vi "Endpoint.vi"(7 "endpointOp":T3, 8 "element in":T4, 10 "parms in":T1={"subchannel"=0, "size (0)"=0, "abort (F)"=FALSE, "timeout"=-1, "ack id (0)"=0, "last elt? (F)"=FALSE, "valid? (T)"=FALSE, "GUID"=""}, 11 "channel in":T5) -> (0 "element out":T4, 2 "parms out":T2)   [LabVIEW 2019, in "MessengerM.lvlib"]
doc: "Reads a message from a MsgPipe Channel (blocks if empty, but not beyond the specified timeout)."
uses:
  <resource>/Channels/MessengerM/MessengerM.lvlib
  <resource>/Channels/MessengerM/ChannelOp.ctl
  <resource>/ChannelSupport/_ChannelSupport/_ChannelSupport.lvlib
  <resource>/Channels/MessengerM/EndpointOp.ctl
  <resource>/Channels/MessengerM/))Channel.ctl
  <resource>/Channels/MessengerM/Element.ctl
  <resource>/Channels/MessengerM/ParmsOut.ctl
  <resource>/Channels/MessengerM/ParmsIn.ctl
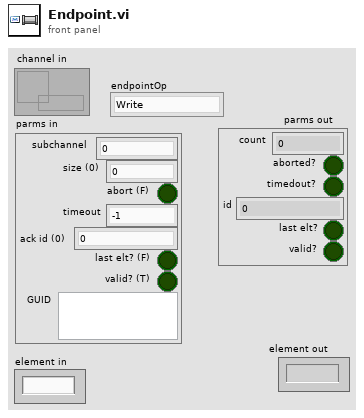
[diagram p1: front panel]
types:
  T1 = typedef "MessengerM.lvlib/ParmsIn.ctl" = cluster{"subchannel":i32, "size (0)":i32, "abort (F)":bool, "timeout":i32, "ack id (0)":u32, "last elt? (F)":bool, "valid? (T)":bool, "GUID":string}
  T2 = typedef "MessengerM.lvlib/ParmsOut.ctl" = cluster{"count":i32, "aborted?":bool, "timedout?":bool, "id":u32, "last elt?":bool, "valid?":bool}
  T3 = typedef "MessengerM.lvlib/EndpointOp.ctl" = enum16{"Write", "WriteAck", "WriteSync", "Read", "ReadAck"}
  T4 = typedef "MessengerM.lvlib/Element.ctl" = string
  T5 = typedef "MessengerM.lvlib/))Channel.ctl" = refnum<queue>
  T6 = typedef "MessengerM.lvlib/ChannelOp.ctl" = enum16{"init", "write", "read", "wreplace", "rreplace", "wrtAck", "rdAck", "rdAck2", "packet", "probe"}
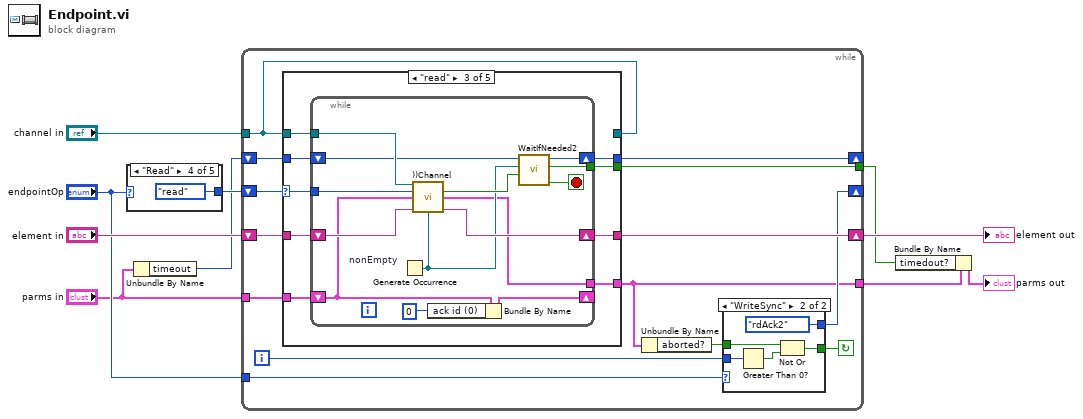
[diagram p0: block diagram]
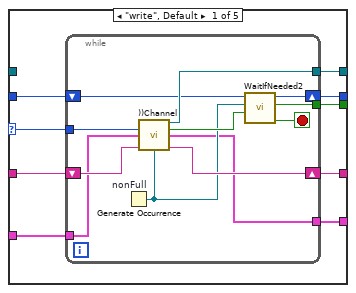
[diagram p2: hidden frame]
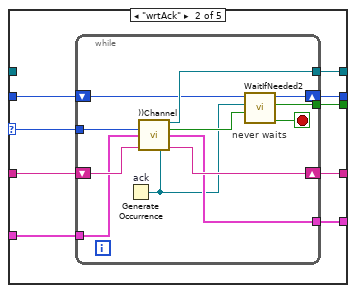
[diagram p3: hidden frame]
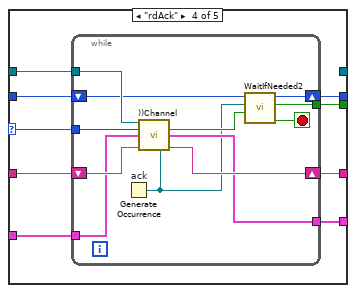
[diagram p4: hidden frame]
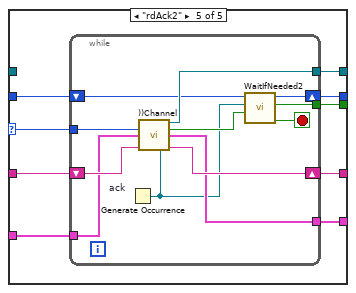
[diagram p5: hidden frame]
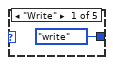
[diagram p7: hidden frame]
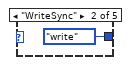
[diagram p8: hidden frame]
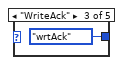
[diagram p9: hidden frame]
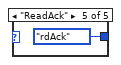
[diagram p10: hidden frame]
diagram:
  n1 = case shown="\"Read\"" "endpointOp" {
    tunnel: [ChannelOp."write" ("channelOp") ChannelOp."write" ("channelOp") ChannelOp."wrtAck" ("channelOp") ChannelOp."read" ("channelOp") ChannelOp."rdAck" ("channelOp")] -> w8
    frame "Write" {
    }
    frame "WriteSync" {
    }
    frame "WriteAck" {
    }
    frame "Read" {
    }
    frame "ReadAck" {
    }
  }
  n2 = Unbundle By Name("parms in") -> ("timeout"=w4:i32)
  n3 = while {
    tunnel: [w28] -> w1
    tunnel: "endpointOp" -> [w21]
    shift-right: [w23] -> _
    shift-left: w8 -> [w25]
    tunnel: "channel in" -> [w20]
    shift-right: [w29] -> w6
    shift-left: "element in" -> [w27]
    tunnel: "parms in" -> [w19]
    shift-right: [w18] -> _
    shift-left: w4 -> [w26]
    tunnel: [w17] -> w3
    i -> [w22]
    stop <- w24 continue-if-true
    n4 = case shown="\"read\"" w25 {
      selector: w25 -> [w34 w55 w76 w99 w120]
      tunnel: [w38 w59 w80 w103 w124] -> w29
      tunnel: [w37 w58 w79 w102 w123] -> w28
      tunnel: w27 -> [w36 w57 w78 w101 w122]
      tunnel: w26 -> [w35 w56 w77 w100 w121]
      tunnel: [w33 w54 _ _ w119] -> w20
      tunnel: w20 -> [_ _ w75 w98 _]
      tunnel: w19 -> [w30 w51 w72 w95 w118]
      tunnel: [w32 w53 w74 w97 w117] -> w18
      tunnel: [w31 w52 w73 w96 w116] -> w17
      frame "write", Default {
        n5 = while {
          tunnel: w34 -> [w49]
          tunnel: [w46] -> w37
          tunnel: [w47] -> w33
          shift-right: [w50] -> w38
          shift-left: w36 -> [w48]
          shift-right: [w41] -> w32
          shift-left: w35 -> [w44]
          tunnel: [w40] -> w31
          tunnel: w30 -> [w39]
          stop <- w45 stop-if-true
          n6 = Generate Occurrence "nonFull"() -> (w42:refnum<k4>)
          n7 = call <resource>:"))Channel.vi"("channelOp"=w49, "parms in"=w39, "element in"=w48, "nonfull/empty"=w42) -> ("channel out"=w47:T5, "wait"=w43:bool, "parms out"=w40:T2, "element out"=w50:T4)  [unwired: 6 in, 2 out]
          n8 = call <resource>:"WaitIfNeeded2.vi"("wait"=w43, "occ"=w42, "_timeout (ms) in"=w44) -> ("stop loop"=w45:bool, "timed out"=w46:bool, "_timeout (ms) out"=w41:i32)  [unwired: 6 in]
        }
      }
      frame "wrtAck" {
        n9 = while {
          tunnel: w55 -> [w70]
          tunnel: [w67] -> w58
          tunnel: [w68] -> w54
          shift-right: [w71] -> w59
          shift-left: w57 -> [w69]
          shift-right: [w63] -> w53
          shift-left: w56 -> [w65]
          tunnel: [w62] -> w52
          tunnel: w51 -> [w61]
          stop <- w66 stop-if-true
          # "never waits"
          n10 = Generate Occurrence "ack"() -> (w60:refnum<k4>)
          n11 = call <resource>:"))Channel.vi"("channelOp"=w70, "parms in"=w61, "element in"=w69, "ackOcc"=w60) -> ("channel out"=w68:T5, "wait"=w64:bool, "parms out"=w62:T2, "element out"=w71:T4)  [unwired: 6 in, 2 out]
          n12 = call <resource>:"WaitIfNeeded2.vi"("wait"=w64, "occ"=w60, "_timeout (ms) in"=w65) -> ("stop loop"=w66:bool, "timed out"=w67:bool, "_timeout (ms) out"=w63:i32)  [unwired: 6 in]
        }
      }
      frame "read" {
        n13 = while {
          tunnel: w76 -> [w93]
          tunnel: [w90] -> w79
          tunnel: w75 -> [w91]
          shift-right: [w94] -> w80
          shift-left: w78 -> [w92]
          shift-right: [w85] -> w74
          shift-left: w77 -> [w88]
          tunnel: [w84] -> w73
          shift-right: [w82] -> _
          shift-left: w72 -> [w83]
          stop <- w89 stop-if-true
          n14 = Generate Occurrence "nonEmpty"() -> (w86:refnum<k4>)
          n15 = call <resource>:"))Channel.vi"("channel in"=w91, "channelOp"=w93, "parms in"=w83, "element in"=w92, "nonfull/empty"=w86) -> ("wait"=w87:bool, "parms out"=w84:T2, "element out"=w94:T4)  [unwired: 5 in, 3 out]
          n16 = Bundle By Name(cluster=w83, "ack id (0)"=u32 0) -> (w82:T1)
          n17 = call <resource>:"WaitIfNeeded2.vi"("wait"=w87, "occ"=w86, "_timeout (ms) in"=w88) -> ("stop loop"=w89:bool, "timed out"=w90:bool, "_timeout (ms) out"=w85:i32)  [unwired: 6 in]
        }
      }
      frame "rdAck" {
        n18 = while {
          tunnel: w99 -> [w114]
          tunnel: [w111] -> w102
          tunnel: w98 -> [w112]
          shift-right: [w115] -> w103
          shift-left: w101 -> [w113]
          shift-right: [w107] -> w97
          shift-left: w100 -> [w109]
          tunnel: [w106] -> w96
          tunnel: w95 -> [w105]
          stop <- w110 stop-if-true
          n19 = Generate Occurrence "ack"() -> (w104:refnum<k4>)
          n20 = call <resource>:"))Channel.vi"("channel in"=w112, "channelOp"=w114, "parms in"=w105, "element in"=w113, "ackOcc"=w104) -> ("wait"=w108:bool, "parms out"=w106:T2, "element out"=w115:T4)  [unwired: 5 in, 3 out]
          n21 = call <resource>:"WaitIfNeeded2.vi"("wait"=w108, "occ"=w104, "_timeout (ms) in"=w109) -> ("stop loop"=w110:bool, "timed out"=w111:bool, "_timeout (ms) out"=w107:i32)  [unwired: 6 in]
        }
      }
      frame "rdAck2" {
        n22 = while {
          tunnel: w120 -> [w135]
          tunnel: [w132] -> w123
          tunnel: [w133] -> w119
          shift-right: [w136] -> w124
          shift-left: w122 -> [w134]
          tunnel: w118 -> [w128]
          shift-right: [w127] -> w117
          shift-left: w121 -> [w130]
          tunnel: [w126] -> w116
          stop <- w131 stop-if-true
          n23 = Generate Occurrence "ack"() -> (w125:refnum<k4>)
          n24 = call <resource>:"))Channel.vi"("channelOp"=w135, "parms in"=w128, "element in"=w134, "ackOcc"=w125) -> ("channel out"=w133:T5, "wait"=w129:bool, "parms out"=w126:T2, "element out"=w136:T4)  [unwired: 6 in, 2 out]
          n25 = call <resource>:"WaitIfNeeded2.vi"("wait"=w129, "occ"=w125, "_timeout (ms) in"=w130) -> ("stop loop"=w131:bool, "timed out"=w132:bool, "_timeout (ms) out"=w127:i32)  [unwired: 6 in]
        }
      }
    }
    n26 = Unbundle By Name(w17) -> ("aborted?"=w16:bool)
    n27 = case shown="\"WriteSync\"" w21 {
      tunnel: [_ ChannelOp."rdAck2" ("channelOp")] -> w23
      tunnel: [_ w140] -> w24
      tunnel: w16 -> [_ w139]
      tunnel: w22 -> [_ w137]
      frame Default {
      }
      frame "WriteSync" {
        n28 = Greater Than 0?(x=w137) -> (x > 0?=w138:bool)
        n29 = Not Or(1:w138, 2:w139) -> (0:w140:bool)
      }
    }
  }
  "element out" <- w6
  n30 = Bundle By Name(cluster=w3, "timedout?"=w1) -> (→"parms out":T2)
